vi "Write outputData.vi"(10 "outputData":T1 {"Step & Direction" min=-32767}, 11 "SendOutputData in":refnum<class "SendOutputData.lvclass">) -> (3 "SendOutputData out":refnum<class "SendOutputData.lvclass">)   [LabVIEW 2013, in "SendOutputData.lvclass"]
uses:
  SendOutputData.lvclass
  <userlib>/Common/ILC/Typedefs/OutputData.ctl
  SendOutputData.lvclass/SendOutputData.ctl
  <userlib>/Common/ILC/Typedefs/ILCTypedefs.lvlib
panel:
  # "DAC"
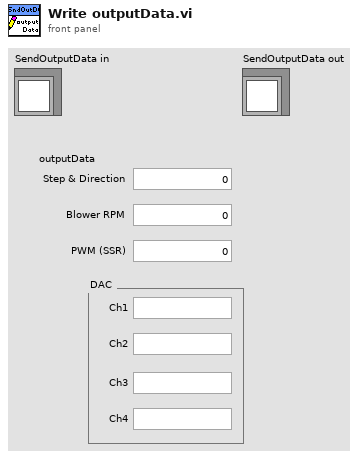
[diagram p1: front panel]
types:
  T1 = typedef "ILCCommon.lvlib/ILCTypedefs.lvlib/OutputData.ctl" = cluster{"Step & Direction":i16, "Blower RPM":u8, "PWM (SSR)":u8, "Ch1":u16, "Ch2":u16, "Ch3":u16, "Ch4":u16}
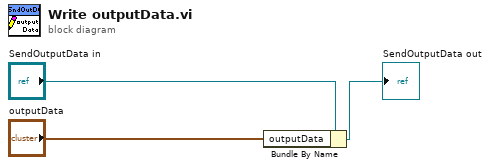
[diagram p0: block diagram]
diagram:
  n1 = Bundle By Name(cluster="SendOutputData in", "outputData"="outputData") -> (→"SendOutputData out":refnum<class "SendOutputData.lvclass">)
